vi "Cash-flow.vi"(1 "Dettes":dbl, 2 "Argent ventes":dbl, 3 "CA":dbl) -> (0 "Cash Flow":dbl)   [LabVIEW 2024]
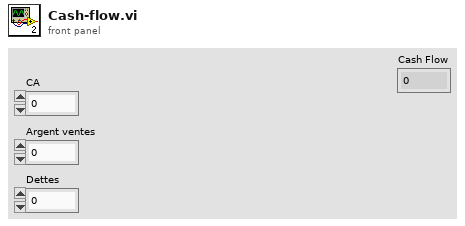
[diagram p1: front panel]
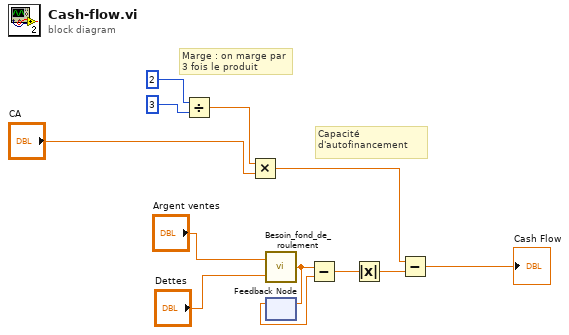
[diagram p0: block diagram]
diagram:
  # "Capacité d'autofinancement"
  # "Marge : on marge par 3 fois le produit"
  n1 = Divide(x=2, y=3) -> (x/y=w4:dbl)
  n2 = Multiply(x=w4, y="CA") -> (x*y=w2:dbl)
  n3 = call "Besoin_fond_de_roulement.vi"("Argent ventes"="Dettes", "dettes"="Argent ventes") -> ("BFR"=w9:dbl)
  n4 = feedback-in #1(w9) -> ()
  n5 = feedback #1() -> (w11:dbl)  [unwired: 1 in]
  n6 = Subtract(x=w9, y=w11) -> (x-y=w12:dbl)
  n7 = Absolute Value(x=w12) -> (abs(x)=w10:dbl)
  n8 = Subtract(x=w2, y=w10) -> (x-y=→"Cash Flow":dbl)
